vi "set_trm_info.vi"(6 "yw":string, 8 "sp_shuoming":string, 9 "sp_yijian":string, 10 "id":string, 11 "lc_num":string) -> (0 "error":errorcluster, 2 "error 2":errorcluster caption="error")   [LabVIEW 2017, in "Lib_code.lvlib"]
uses:
  Lib_code.lvlib
panel:
  in  "error 4":errorcluster={"status"=TRUE, "code"=254, "source"="您无权申请该流程！"} caption="error"
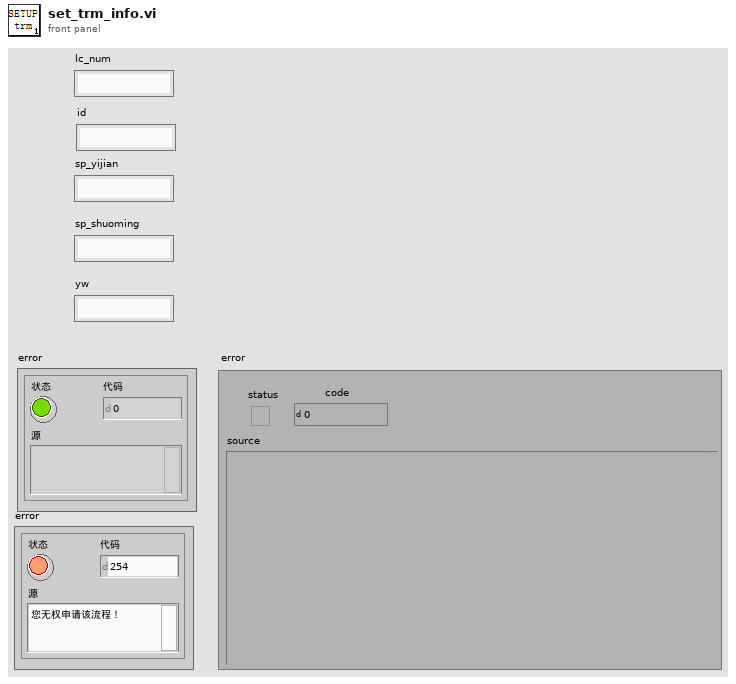
[diagram p1: front panel]
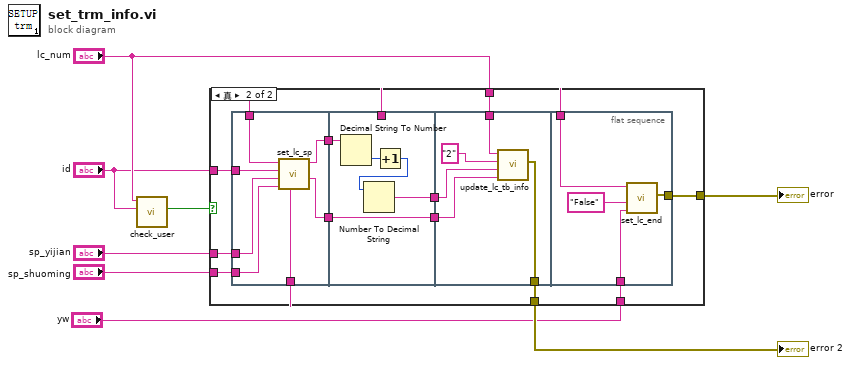
[diagram p0: block diagram]
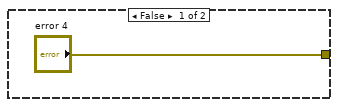
[diagram p2: hidden frame]
diagram:
  n1 = call "check_user.vi"("id"="id", "lc_num"="lc_num") -> ("check"=w1:bool)  [unwired: 8 in, 1 out]
  n2 = case shown="真" w1 {
    tunnel: "sp_yijian" -> [_ w16]
    tunnel: "sp_shuoming" -> [_ w15]
    tunnel: ["error 4" w14] -> w6
    tunnel: [_ w13] -> w5
    tunnel: "yw" -> [_ w12]
    tunnel: "lc_num" -> [_ w11]
    tunnel: "id" -> [_ w10]
    frame False {
    }
    frame True {
      n3 = flat-sequence {
        tunnel: [w27] -> w20
        tunnel: [w26] -> w19
        tunnel: w11 -> [w25]
        tunnel: w10 -> [w24]
        tunnel: w16 -> [w23]
        tunnel: w15 -> [w22]
        tunnel: w12 -> [w21]
        tunnel: w20 -> [w32]
        tunnel: [w29] -> w18
        tunnel: w19 -> [w28]
        tunnel: [w28] -> w17
        tunnel: w11 -> [_]
        tunnel: w18 -> [w35]
        tunnel: w17 -> [w34]
        tunnel: w11 -> [w37]
        tunnel: [w33] -> w13
        tunnel: w11 -> [w39]
        tunnel: w12 -> [w38]
        tunnel: [w40] -> w14
        frame #0 {
          n4 = call "set_lc_sp.vi"("yw"=w21, "sp_shuoming"=w22, "sp_yijian"=w23, "id"=w24, "lc_num"=w25) -> ("cur_spnum"=w26:string, "cur_spsta"=w27:string)  [unwired: 4 in, 1 out]
        }
        frame #1 {
          n5 = Decimal String To Number(string=w32) -> (number=w31:i32)  [unwired: 2 in, 1 out]
          n6 = Increment(x=w31) -> (x+1=w30:i32)
          n7 = Number To Decimal String(number=w30) -> (decimal integer string=w29:string)  [unwired: 1 in]
        }
        frame #2 {
          n8 = call "update_lc_tb_info.vi"("cur_spnum"=w34, "nx_spsta"=w35, "nx_spren"="2", "lc_num"=w37) -> ("error"=w33:errorcluster)  [unwired: 7 in]
        }
        frame #3 {
          n9 = call "set_lc_end.vi"("yw"=w38, "state"="False", "lc_num"=w39) -> ("error"=w40:errorcluster)  [unwired: 8 in]
        }
      }
    }
  }
  "error" <- w6
  "error 2" <- w5
